vi "Drive SS Outputs.vi"(11 "Drive SS Actuator Values In":T1) -> ()   [LabVIEW 2014]
uses:
  Drive SS Actuator Values.ctl
  Global Variables/Refnum Names.vi
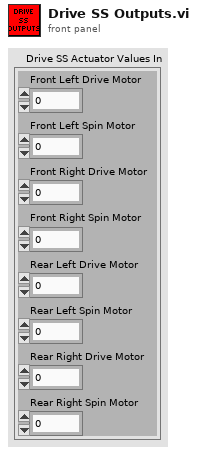
[diagram p1: front panel]
types:
  T1 = typedef "Drive SS Actuator Values.ctl" = cluster{"Front Left Drive Motor":dbl, "Front Left Spin Motor":dbl, "Front Right Drive Motor":dbl, "Front Right Spin Motor":dbl, "Rear Left Drive Motor":dbl, "Rear Left Spin Motor":dbl, "Rear Right Drive Motor":dbl, "Rear Right Spin Motor":dbl}
  T2 = typedef "WPI_MotorControlDeviceRef.ctl" = cluster{"DeviceStatus":errorcluster, "Type":T3, "PWM":cluster{"Controller":T4, "PWM Channel":T5, "DeadBand":T6}, "CAN":cluster{"Device Number":u8, "Control Mode":T7, "Semaphore":T8, "Max Vout":dbl, "TalonSRX Control Mode":T9}, "Invert":bool, "TransformRef":T10, "InvTransformRef":T10}
  T3 = typedef "WPI_MotorControlType.ctl" = enum16{"PWM", "CAN", "CANTalonSRX"}
  T4 = typedef "FPGA_TypedefDigitalModule.ctl" = enum16{"Controller 1"}
  T5 = typedef "FPGA_DIOPWMChannel.ctl" = enum8{"PWM 0", "PWM 1", "PWM 2", "PWM 3", "PWM 4", "PWM 5", "PWM 6", "PWM 7", "PWM 8", "PWM 9", "PWM MXP 0", "PWM MXP 1", "PWM MXP 2", "PWM MXP 3", "PWM MXP 4", "PWM MXP 5", "PWM MXP 6", "PWM MXP 7", "PWM MXP 8", "PWM MXP 9", "Invalid"}
  T6 = typedef "WPI_PWMDeadband.ctl" = cluster{"Name":string, "maxPositivePwm":i32, "minPositivePwm":i32, "centerPwm":i32, "maxNegativePwm":i32, "minNegativePwm":i32, "angularRange":u16}
  T7 = typedef "WPI_CANJaguar_ControlMode.ctl" = enum8{"Percent VBus", "Current", "Speed", "Position", "Voltage"}
  T8 = typedef "Semaphore RefNum" = refnum<k1>
  T9 = typedef "WPI_CANTalonSRX_APIControlMode.ctl" = enum8{"Percent VBus", "Speed", "Position", "Slave", "Unchanged / Invalid"}
  T10 = typedef "WPI_PWMTransform_ConPane.ctl" = refnum<vi>
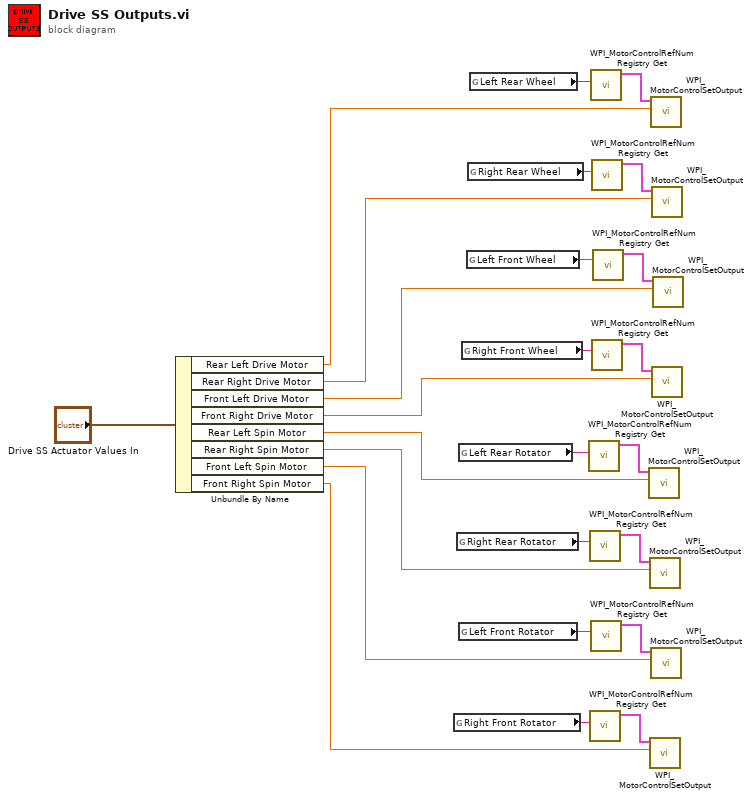
[diagram p0: block diagram]
diagram:
  n1 = Unbundle By Name("Drive SS Actuator Values In") -> ("Rear Left Drive Motor"=w16:dbl, "Rear Right Drive Motor"=w15:dbl, "Front Left Drive Motor"=w14:dbl, "Front Right Drive Motor"=w13:dbl, "Rear Left Spin Motor"=w12:dbl, "Rear Right Spin Motor"=w9:dbl, "Front Left Spin Motor"=w10:dbl, "Front Right Spin Motor"=w11:dbl)
  n2 = global read "Refnum Names.vi" "Right Front Rotator"() -> (w1:string)
  n3 = global read "Refnum Names.vi" "Right Rear Rotator"() -> (w3:string)
  n4 = global read "Refnum Names.vi" "Left Rear Rotator"() -> (w4:string)
  n5 = global read "Refnum Names.vi" "Left Front Rotator"() -> (w2:string)
  n6 = global read "Refnum Names.vi" "Right Front Wheel"() -> (w5:string)
  n7 = global read "Refnum Names.vi" "Left Front Wheel"() -> (w6:string)
  n8 = global read "Refnum Names.vi" "Right Rear Wheel"() -> (w7:string)
  n9 = global read "Refnum Names.vi" "Left Rear Wheel"() -> (w8:string)
  n10 = call <vilib>:"WPI_MotorControlRefNum Registry Get.vi"("refnum name"=w4) -> ("MotorControlDevRef"=w21:T2)  [unwired: 9 in, 1 out]
  n11 = call <vilib>:"WPI_MotorControlRefNum Registry Get.vi"("refnum name"=w3) -> ("MotorControlDevRef"=w20:T2)  [unwired: 9 in, 1 out]
  n12 = call <vilib>:"WPI_MotorControlRefNum Registry Get.vi"("refnum name"=w1) -> ("MotorControlDevRef"=w18:T2)  [unwired: 9 in, 1 out]
  n13 = call <vilib>:"WPI_MotorControlRefNum Registry Get.vi"("refnum name"=w8) -> ("MotorControlDevRef"=w22:T2)  [unwired: 9 in, 1 out]
  n14 = call <vilib>:"WPI_MotorControlRefNum Registry Get.vi"("refnum name"=w2) -> ("MotorControlDevRef"=w19:T2)  [unwired: 9 in, 1 out]
  n15 = call <vilib>:"WPI_MotorControlRefNum Registry Get.vi"("refnum name"=w7) -> ("MotorControlDevRef"=w23:T2)  [unwired: 9 in, 1 out]
  n16 = call <vilib>:"WPI_MotorControlRefNum Registry Get.vi"("refnum name"=w5) -> ("MotorControlDevRef"=w25:T2)  [unwired: 9 in, 1 out]
  n17 = call <vilib>:"WPI_MotorControlRefNum Registry Get.vi"("refnum name"=w6) -> ("MotorControlDevRef"=w24:T2)  [unwired: 9 in, 1 out]
  n18 = call <vilib>:"WPI_MotorControlSetOutput.vi"("Output"=w12, "MotorControlDevRef"=w21) -> ()  [unwired: 7 in, 3 out]
  n19 = call <vilib>:"WPI_MotorControlSetOutput.vi"("Output"=w9, "MotorControlDevRef"=w20) -> ()  [unwired: 7 in, 3 out]
  n20 = call <vilib>:"WPI_MotorControlSetOutput.vi"("Output"=w11, "MotorControlDevRef"=w18) -> ()  [unwired: 7 in, 3 out]
  n21 = call <vilib>:"WPI_MotorControlSetOutput.vi"("Output"=w16, "MotorControlDevRef"=w22) -> ()  [unwired: 7 in, 3 out]
  n22 = call <vilib>:"WPI_MotorControlSetOutput.vi"("Output"=w10, "MotorControlDevRef"=w19) -> ()  [unwired: 7 in, 3 out]
  n23 = call <vilib>:"WPI_MotorControlSetOutput.vi"("Output"=w15, "MotorControlDevRef"=w23) -> ()  [unwired: 7 in, 3 out]
  n24 = call <vilib>:"WPI_MotorControlSetOutput.vi"("Output"=w13, "MotorControlDevRef"=w25) -> ()  [unwired: 7 in, 3 out]
  n25 = call <vilib>:"WPI_MotorControlSetOutput.vi"("Output"=w14, "MotorControlDevRef"=w24) -> ()  [unwired: 7 in, 3 out]
